vi "LED Matrix Origin.vi"(8 "error in (no error)":errorcluster, 11 "Refnum in":refnum<k20>) -> (0 "error out":errorcluster, 3 "Refnum out":refnum<k20>)   [LabVIEW 2013]
uses:
  <vilib>/rvi/interface/common/niFpgaWaitOnOcc.vi
  <vilib>/Utility/error.llb/Error Cluster From Error Code.vi
  <vilib>/rvi/errors/niLvFpgaAdjustHostInterfaceError.vi
  <vilib>/rvi/interface/nirviReadWriteControl/nirviReadWriteControl.xnode
  NiFpgaLv.dll
  <vilib>/rvi/interface/Simulation/niFpgaSimulationCallBeginRW.vi
panel:
  # "For now, leave Height & Width as internal constants.\nHowever, it would be trivial to make them controls."
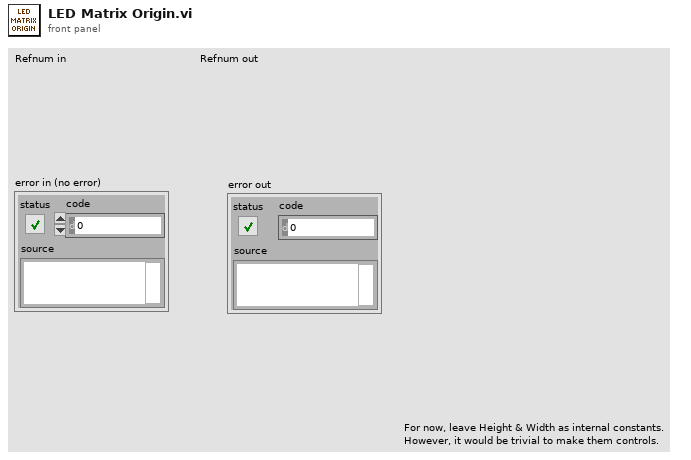
[diagram p1: front panel]
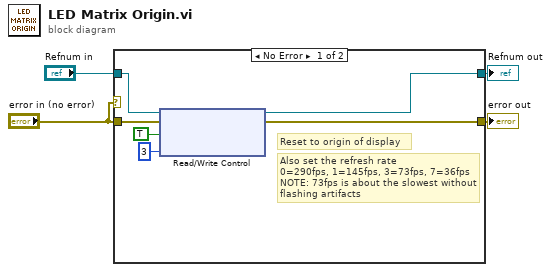
[diagram p0: block diagram]
diagram:
  n1 = case shown="No Error" "error in (no error)" {
    tunnel: [w7 w12] -> w4
    tunnel: "error in (no error)" -> [w9 w11]
    tunnel: "Refnum in" -> [w10 w12]
    tunnel: [w6 w11] -> w2
    frame No Error {
      # "Also set the refresh rate\n0=290fps, 1=145fps, 3=73fps, 7=36fps\nNOTE: 73fps is about the slowest without flashing artifacts"
      # "Reset to origin of display"
      n2 = xnode "Read/Write Control"("FPGA VI Reference In"=w10, "error in"=w9, "LEDMatrix.origin"=TRUE, "LEDMatrix.clkdiv"=u8 3 ("LEDMatrix.rate")) -> ("FPGA VI Reference Out"=w7:refnum<k20>, "error out"=w6:errorcluster)
    }
    frame Error {
    }
  }
  "Refnum out" <- w4
  "error out" <- w2
